vi "force_et_angle_Joy.vi"(10 "axe 1":dbl, 11 "axe 2":dbl) -> (2 "angle":dbl, 3 "in_dead_zone":bool, 5 "force":dbl)   [LabVIEW 2015]
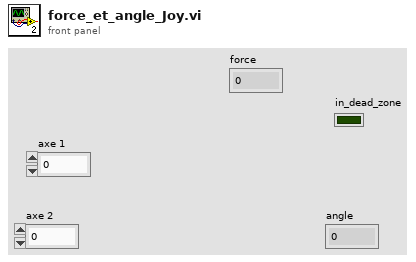
[diagram p1: front panel]
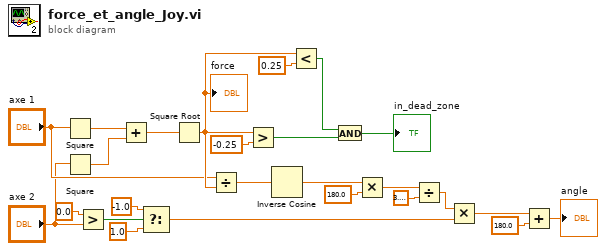
[diagram p0: block diagram]
diagram:
  n1 = Square(x="axe 1") -> (x^2=w24:dbl)
  n2 = Square(x="axe 2") -> (x^2=w25:dbl)
  n3 = Greater?(x=0.0, y="axe 2") -> (0:w16:bool)
  n4 = Add(x=w24, y=w25) -> (x+y=w23:dbl)
  n5 = Select(t=-1.0, s=w16, f=1.0) -> (s? t:f=w14:dbl)
  n6 = Square Root(x=w23) -> (sqrt(x)=w7:dbl)
  "force" <- w7
  n7 = Divide(x="axe 1", y=w7) -> (x/y=w22:dbl)
  n8 = Greater?(x=w7, y=-0.25) -> (0:w5:bool)
  n9 = Inverse Cosine(1:w22) -> (0:w17:dbl)
  n10 = Less?(x=w7, y=0.25) -> (x < y?=w6:bool)
  n11 = And(x=w6, y=w5) -> (x .and. y?=→"in_dead_zone":bool)
  n12 = Multiply(x=w17, y=180.0) -> (x*y=w20:dbl)
  n13 = Divide(x=w20, y=3.141592653589793) -> (x/y=w11:dbl)
  n14 = Multiply(x=w11, y=w14) -> (x*y=w13:dbl)
  n15 = Add(x=w13, y=180.0) -> (x+y=→"angle":dbl)
